vi "RunTest.vi"(8 "error in":errorcluster, 11 "Prueba31 in":refnum<class "Prueba32.lvclass">) -> (0 "error out":errorcluster, 2 "Resultado":string, 3 "Prueba31 out":refnum<class "Prueba32.lvclass">)   [LabVIEW 2019, in "Prueba32.lvclass"]
uses:
  Prueba32.lvclass
  Prueba32.lvclass/Prueba32.ctl
  <vilib>/Utility/miscctls.llb/LVRowAndColumnTypeDef.ctl
  QMH/Message Queue/Enqueue Message (Single).vi
  <vilib>/Utility/error.llb/Error Cluster From Error Code.vi
  RerenceAllControlsToolkit/_get control reference by name.vi
  <vilib>/ErrorRing/Error Ring.xnode
  QMH/Message Queue/Message Queue.lvlib
  QMH/User Event - Stop/User Event - Stop.lvlib
panel:
  in  "Tab":enum32{"externo", "interno"}(tab)
  out "Pict RingB_Ext":u16(ring)
  out "curva_referencia_Ext":dbl
  in  "cb_frec_Ext":string(combo)="63"
  in  "boton_generar_Ext":bool
  out "cumple_Ext":bool
  out "no_cumple_Ext":bool
  in  "seguir_Ext":bool
  out "voltaje_Ext":dbl format="%_3f"
  out "frecuencia_Ext":dbl format="%.2f"
  out "tipo generador_Ext":string
  out "Pict RingA_Ext":u16(ring)
  in  "Tabla_Ext":string[][](table)=[["63"], ["125"], ["250"], ["500"], ["1000"], ["2000"], ["4000"], ["8000"]]
  out "cumple_Int":bool
  out "no_cumple_Int":bool
  in  "seguir_Int":bool
  out "tipo generador_Int":string
  out "Pict RingA_Int":u16(ring)
  out "Pict RingB_Int":u16(ring)
  in  "Tabla_Int":string[][](table)
  # "Cumple"
  # "No Cumple"
  # "Curva de Referencia"
  # "Frecuencia"
  # "2. Ponderación frecuencial A (entrada acústica). IEC 61252: 2002 Cláusula 7"
  # "Monitoreo"
  # "Frecuencia"
  # "Hz"
  # "Voltaje"
  # "V"
  # "Cumple"
  # "No Cumple"
  # "2. Ponderación frecuencial A (entrada acústica). IEC 61252: 2002 Cláusula 7"
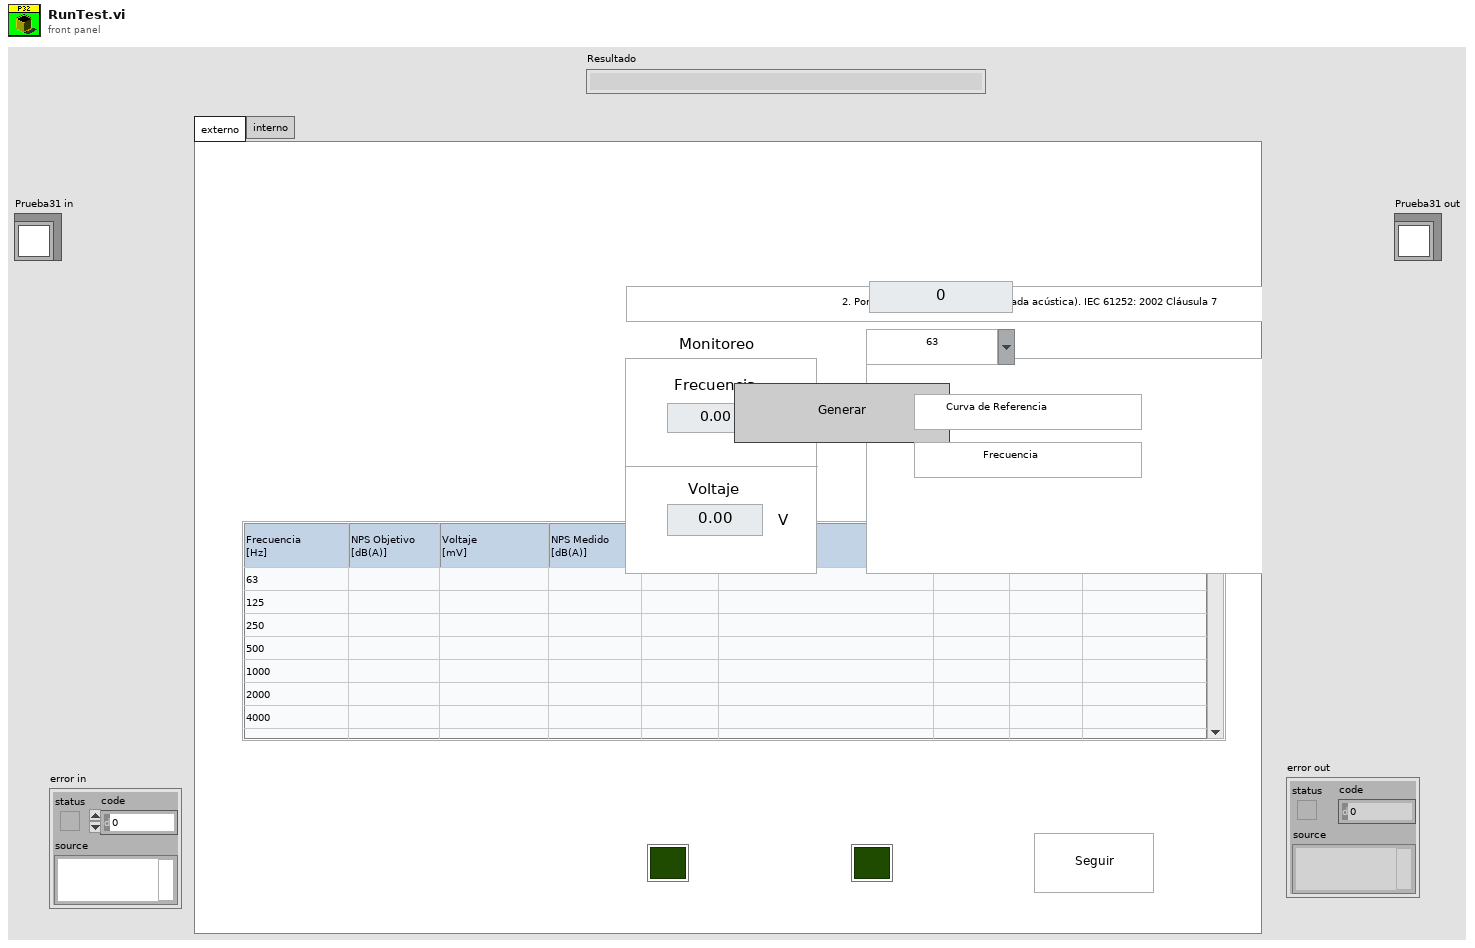
[diagram p1: front panel]
types:
  T1 = typedef "Message Queue.lvlib/All Message Queues.ctl" = cluster{"MHL":refnum<queue>, "Inst_CNT90":refnum<queue>, "Inst_DS360":refnum<queue>, "Inst_Keithley2002":refnum<queue>, "Inst_DAQ":refnum<queue>, "BD":refnum<queue>, "Pistofono":refnum<queue>, "Nexus":refnum<queue>}
  T2 = typedef "LVRowAndColumnTypeDef.ctl" = cluster{"Row":i32, "Column":i32}
  T3 = cluster{"ControlName":string, "ControlReference":refnum<vi>}[]
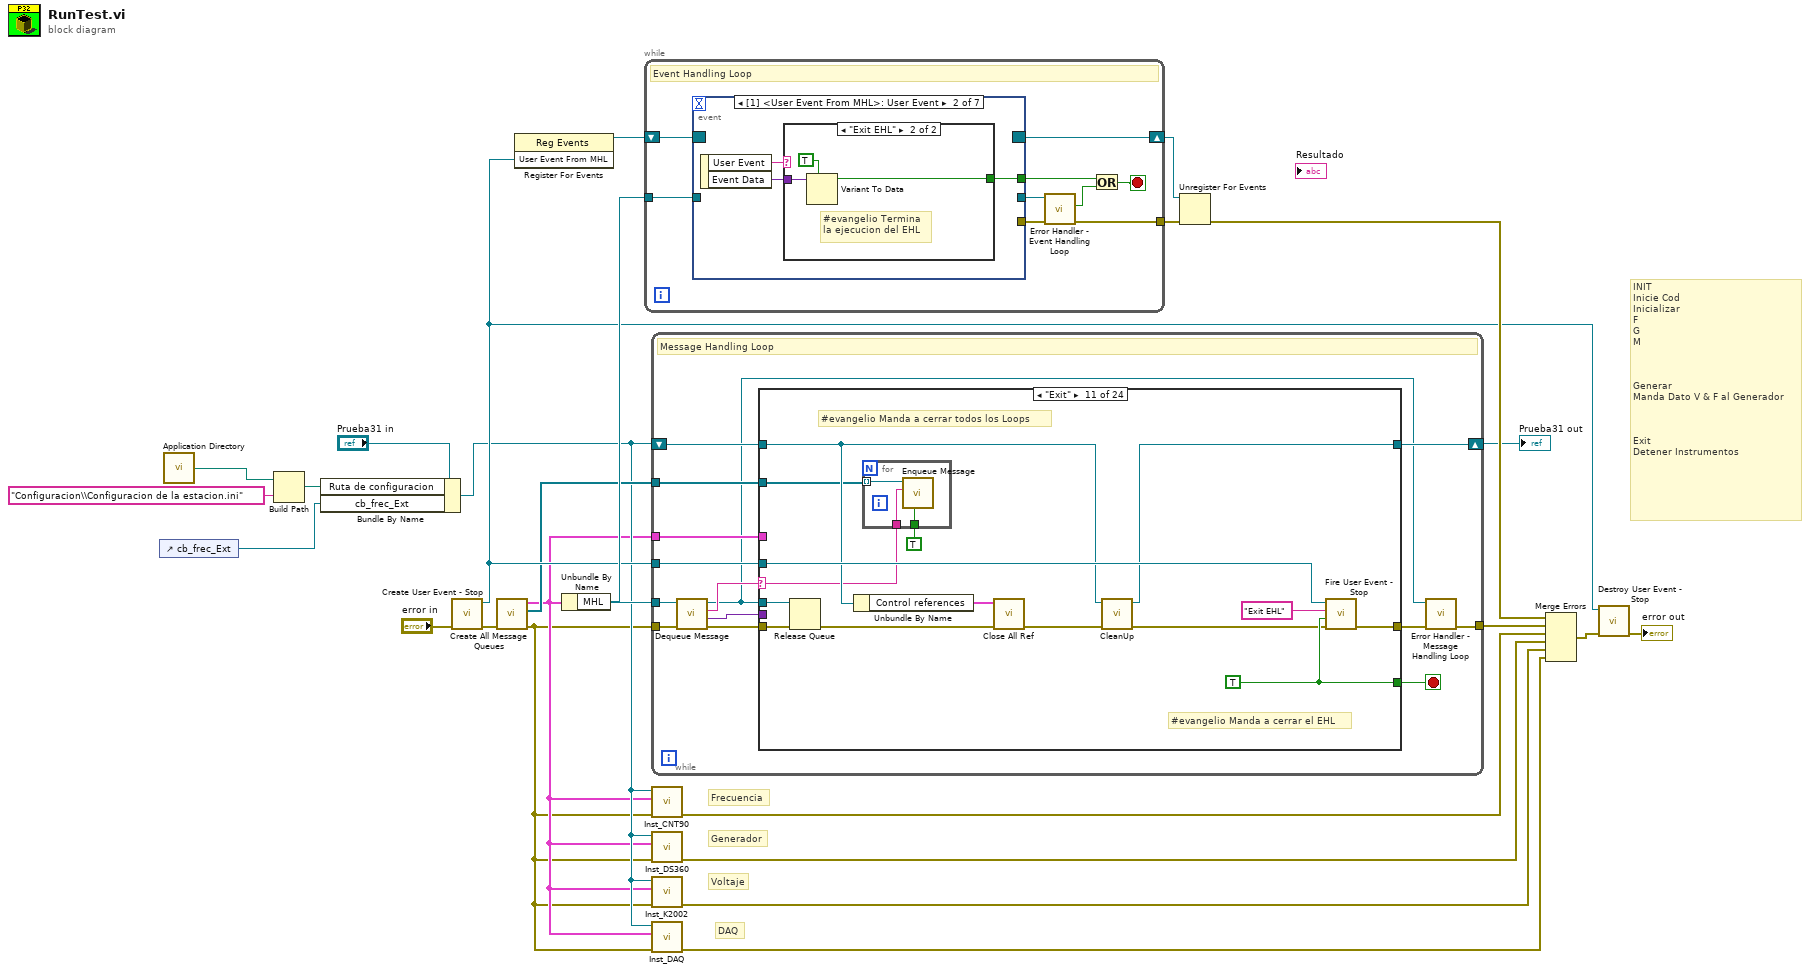
[diagram p0: block diagram]
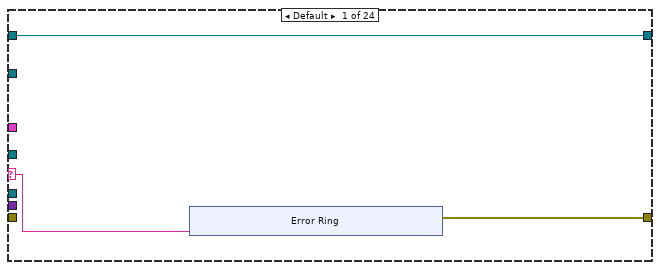
[diagram p2: hidden frame]
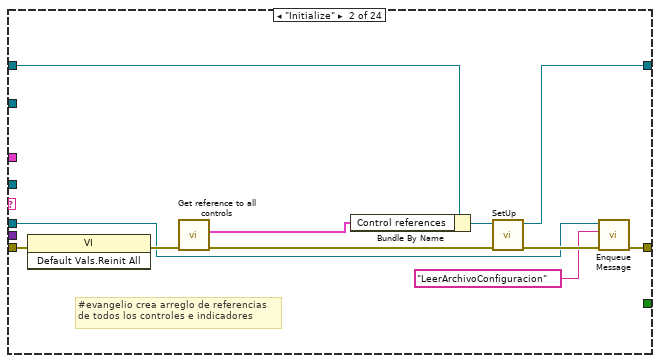
[diagram p3: hidden frame]
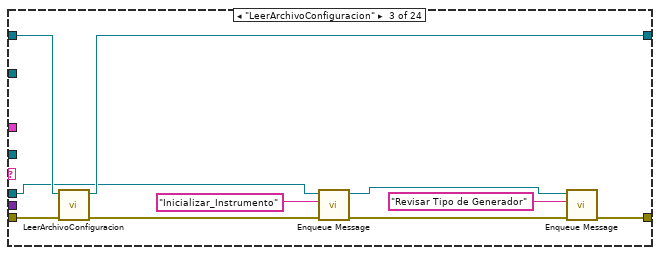
[diagram p4: hidden frame]
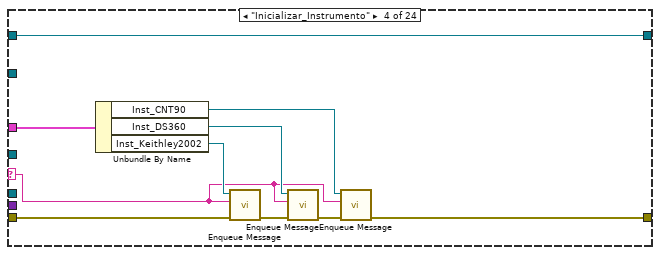
[diagram p5: hidden frame]
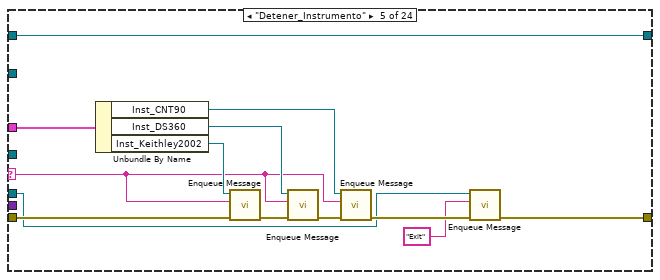
[diagram p6: hidden frame]
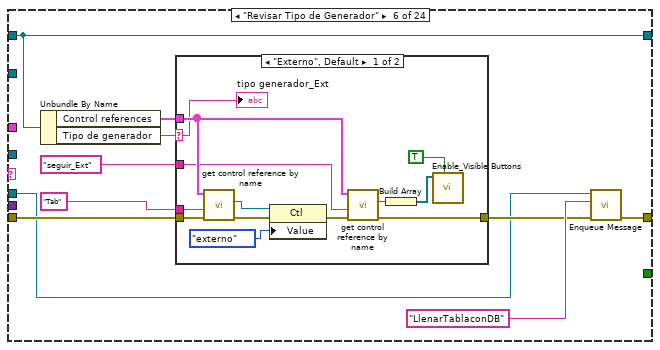
[diagram p7: hidden frame]
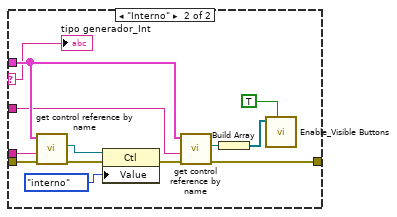
[diagram p8: hidden frame]
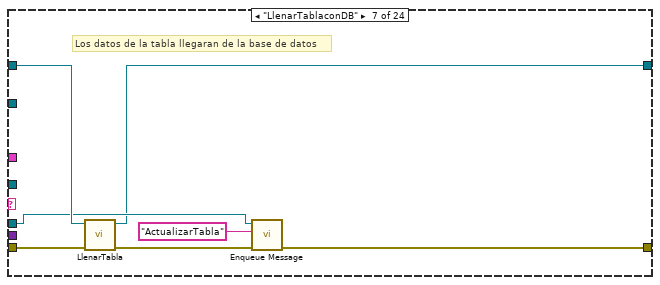
[diagram p9: hidden frame]
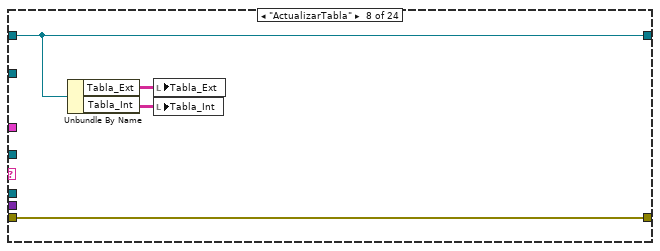
[diagram p10: hidden frame]
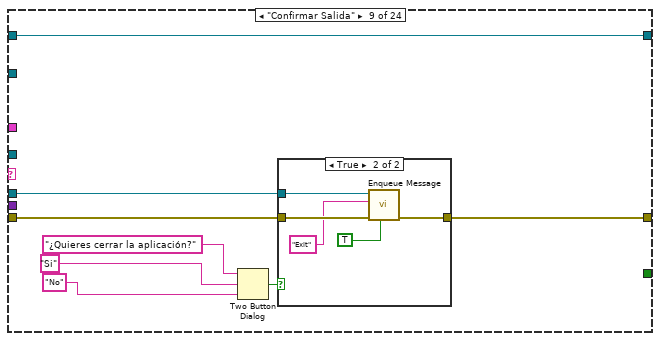
[diagram p11: hidden frame]
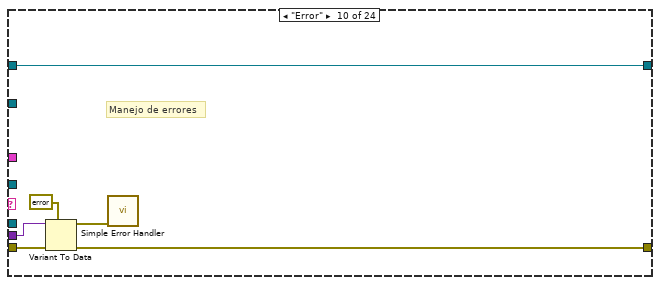
[diagram p13: hidden frame]
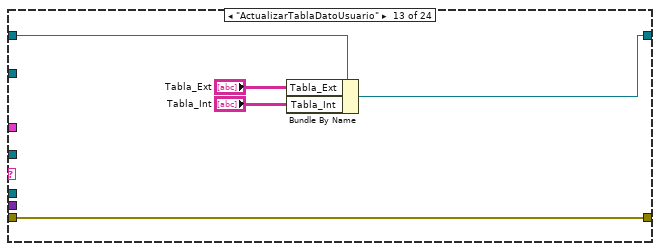
[diagram p15: hidden frame]
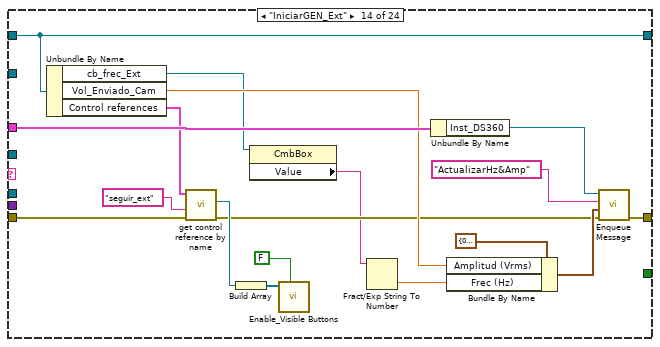
[diagram p16: hidden frame]
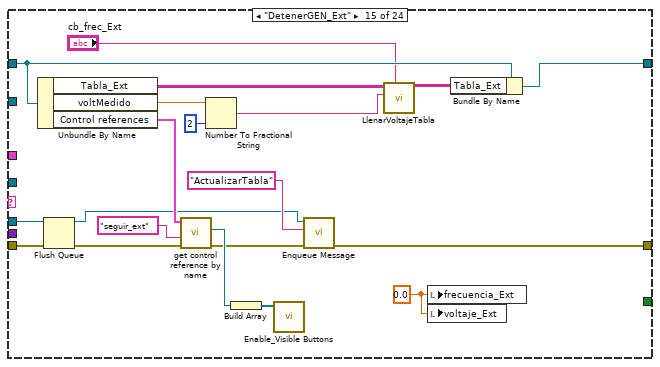
[diagram p17: hidden frame]
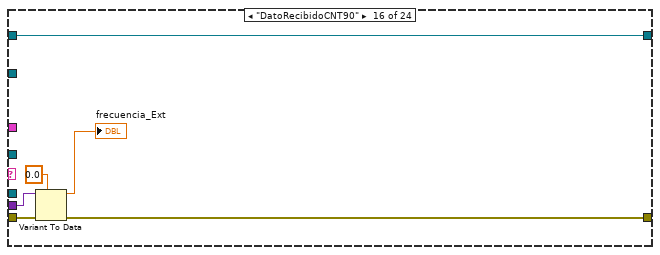
[diagram p18: hidden frame]
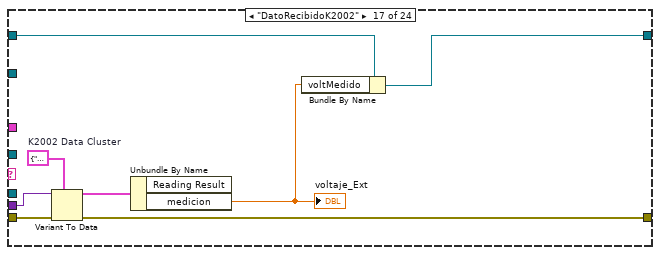
[diagram p19: hidden frame]
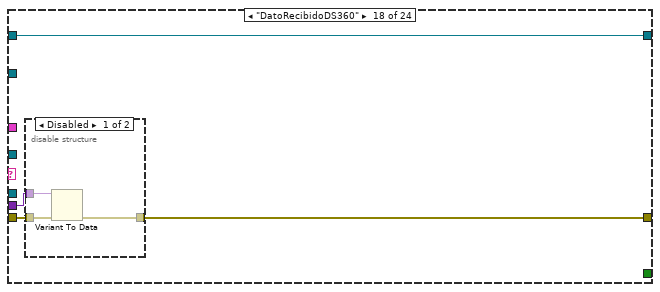
[diagram p20: hidden frame]
diagram:
  # "INIT\nInicie Cod\nInicializar\nF\nG\nM\n\n\n\nGenerar\nManda Dato V & F al Generador\n\n\n\nExit\nDetener Instrumentos"
  # "DAQ"
  # "Generador"
  # "Voltaje"
  # "Frecuencia"
  n1 = control-ref of="cb_frec_Ext"() -> (w1:refnum<vi>)
  n2 = call <vilib>:"Application Directory.vi"() -> ("Application Directory"=w9:path)
  n3 = Build Path(base path=w9, name or relative path="Configuracion\\Configuracion de la estacion.ini") -> (appended path=w8:path)
  n4 = Bundle By Name(cluster="Prueba31 in", "Ruta de configuracion"=w8, "cb_frec_Ext"=w1) -> (w5:refnum<class "Prueba32.lvclass">)
  n5 = call "Create User Event - Stop.vi"("error in (no error)"="error in") -> ("error out"=w22:errorcluster, "User Event From MHL"=w16:refnum<user-event>)  [unwired: 9 in]
  n6 = call "Create All Message Queues.vi"("error in (no error)"=w22) -> ("error out"=w3:errorcluster, "PL Queues Array"=w6:refnum<queue>[], "All Message Queues out"=w4:T1)  [unwired: 8 in]
  n7 = register-events(w16) -> (reference out=w25:refnum<event-registration>)  [unwired: 2 in, 1 out]
  n8 = Unbundle By Name(w4) -> ("MHL"=w21:refnum<queue>)
  n9 = while {
    tunnel: w21 -> [w34]
    tunnel: [w30] -> w24
    shift-right: [w32] -> w23
    shift-left: w25 -> [w33]
    stop <- w26 stop-if-true
    # "Event Handling Loop"
    n10 = event shown="[1] <User Event From MHL>: User Event" {
      selector: w33 -> [_ _ _ _ _ _ _]
      dyn-events: [_ _ _ _ _ _ _] -> w32
      timeout: _ -> [_ _ _ _ _ _ _]
      tunnel: w34 -> [w37 _ w47 w54 w58 w68 w71]
      tunnel: [w39 _ w48 w56 w63 w69 w72] -> w31
      tunnel: [w38 _ _ _ _ _ _] -> w29
      tunnel: [_ w40 _ _ _ _ _] -> w27
      event Panel Close? {
        w35 = TRUE
        n11 = event-data() -> ()  [unwired: 1 in, 1 out]
        n12 = call-poly "Enqueue Message.vi"("Priority Message? (F)"=w35, "Message"="Confirmar Salida", "Message Queue"=w37) -> ("error out"=w39:errorcluster, "dup Message Queue"=w38:refnum<queue>)  [unwired: 7 in]
        n13 = event-data("Discard?"=w35) -> ()  [unwired: 1 in, 1 out]
      }
      event User Event {
        n14 = event-data() -> ("User Event"=w42:string, "Event Data"=w41:variant)  [unwired: 1 in]
        n15 = case shown="\"Exit EHL\"" w42 {
          tunnel: w41 -> [_ w44]
          tunnel: [_ w43] -> w40
          frame Default {
          }
          frame "Exit EHL" {
            # "#evangelio Termina\nla ejecucion del EHL"
            n16 = Variant To Data(type=TRUE, Variant=w44) -> (data=w43:bool)  [unwired: 1 in, 1 out]
          }
        }
      }
      event "seguir_Ext", "seguir_Int": Value Change {
        n17 = event-data() -> ()  [unwired: 1 in, 1 out]
        n18 = call-poly "Enqueue Message.vi"("Message"="Detener_Instrumento", "Message Queue"=w47) -> ("error out"=w48:errorcluster)  [unwired: 8 in, 1 out]
      }
      event "Tabla_Ext": Value Change {
        n19 = event-data() -> ("CtlRef"=w50:refnum<vi>)  [unwired: 1 in]
        n20 = property class="Tbl (strict)"(reference=w50) -> ("Selection Start"=w49:T2)  [unwired: 1 in, 2 out]
        n21 = call-poly "Enqueue Message.vi"("Message"="ActualizarTablaDatoUsuario", "Message Queue"=w54) -> ("error out"=w51:errorcluster, "dup Message Queue"=w53:refnum<queue>)  [unwired: 8 in]
        n22 = call-poly "Enqueue Message.vi"("error in (no error)"=w51, "Message Data"=w49, "Message"="Evaluacion", "Message Queue"=w53) -> ("error out"=w56:errorcluster)  [unwired: 6 in, 1 out]
      }
      event "Tabla_Int": Value Change {
        n23 = event-data() -> ()  [unwired: 1 in, 2 out]
        n24 = property on="Tabla_Int" class="Tbl (strict)"() -> ("Selection Start"=w61:T2)  [unwired: 2 in, 2 out]
        n25 = call-poly "Enqueue Message.vi"("Message"="ActualizarTablaDatoUsuario", "Message Queue"=w58) -> ("error out"=w60:errorcluster, "dup Message Queue"=w59:refnum<queue>)  [unwired: 8 in]
        n26 = call-poly "Enqueue Message.vi"("error in (no error)"=w60, "Message Data"=w61, "Message"="Evaluacion", "Message Queue"=w59) -> ("error out"=w63:errorcluster)  [unwired: 6 in, 1 out]
      }
      event "boton_generar_Ext": Value Change {
        n27 = event-data() -> ()  [unwired: 1 in, 1 out]
        n28 = Select(t="IniciarGEN_Ext" ("Message"), s="boton_generar_Ext", f="DetenerGEN_Ext" ("Message")) -> (s? t:f=w66:string)
        n29 = call-poly "Enqueue Message.vi"("Message"=w66, "Message Queue"=w68) -> ("error out"=w69:errorcluster)  [unwired: 8 in, 1 out]
      }
      event "cb_frec_Ext": Value Change {
        n30 = event-data() -> ()  [unwired: 1 in, 1 out]
        n31 = call-poly "Enqueue Message.vi"("Message"="ActualizarCurvaRef", "Message Queue"=w71) -> ("error out"=w72:errorcluster)  [unwired: 8 in, 1 out]
      }
    }
    n32 = call "Error Handler - Event Handling Loop.vi"("error in (no error)"=w31, "Message Queue"=w29) -> ("dup error in"=w30:errorcluster, "Error?"=w28:bool)  [unwired: 7 in, 1 out]
    n33 = Or(x=w27, y=w28) -> (x .or. y?=w26:bool)
  }
  n34 = while {
    tunnel: w3 -> [w86]
    tunnel: w21 -> [w85]
    tunnel: [w80] -> w19
    shift-right: [w78] -> w17
    shift-left: w5 -> [w79]
    tunnel: w4 -> [w76]
    tunnel: w16 -> [w75]
    tunnel: w6 -> [w74]
    stop <- w77 stop-if-true
    # "Message Handling Loop"
    n35 = call "Dequeue Message.vi"("error in (no error)"=w86, "Message Queue"=w85) -> ("error out"=w82:errorcluster, "Message Data"=w83:variant, "Message"=w84:string, "dup Message Queue"=w73:refnum<queue>)  [unwired: 6 in]
    n36 = case shown="\"Exit\"" w84 {
      selector: w84 -> [w88 _ _ w121 w134 _ _ _ _ _ w210 _ _ _ _ _ _ _ w293 w303 _ _ _ _]
      tunnel: w73 -> [_ w100 w113 _ w129 w141 w180 _ w188 _ w221 _ _ _ w253 _ _ _ _ _ w316 _ _ _]
      tunnel: w83 -> [_ _ _ _ _ _ _ _ _ w203 _ _ _ _ _ w273 w282 w285 w300 w310 w325 _ _ _]
      tunnel: w82 -> [_ w107 w117 w126 w139 w147 w183 w187 w194 w204 w220 w227 w232 w243 w255 w274 w283 w286 w301 w311 w326 w335 w337 w339]
      tunnel: [w87 w101 w108 w118 w130 w142 w177 w187 w193 w205 w218 w227 w232 w241 w251 w275 w284 w287 w297 w307 w317 w335 w337 w339] -> w81
      tunnel: w79 -> [w89 w105 w116 w127 w140 w146 w182 w186 w195 w207 w211 w226 w230 w244 w262 w276 w277 w288 w302 w312 w321 w334 w336 w338]
      tunnel: [w89 w103 w115 w127 w140 w146 w178 w186 w195 w207 w212 w226 w231 w244 w263 w276 w278 w288 w302 w312 w314 w334 w336 w338] -> w78
      tunnel: [_ _ _ _ _ _ _ _ _ _ w215 _ _ _ _ _ _ _ _ _ _ _ _ _] -> w77
      tunnel: w76 -> [_ _ _ w125 w138 _ _ _ _ _ _ _ _ w250 _ _ _ _ w295 w305 _ _ _ _]
      tunnel: w75 -> [_ _ _ _ _ _ _ _ _ _ w217 _ _ _ _ _ _ _ _ _ _ _ _ _]
      tunnel: w74 -> [_ _ _ _ _ _ _ _ _ _ w208 _ _ _ _ _ _ _ _ _ _ _ _ _]
      frame Default {
        n37 = xnode "Error Ring"("parameter 0"=w88) -> ("error out"=w87:errorcluster)
      }
      frame "Initialize" {
        # "#evangelio crea arreglo de referencias\nde todos los controles e indicadores"
        n38 = invoke class="VI" method="Default Vals.Reinit All"(error in=w107) -> (error out=w106:errorcluster)  [unwired: 2 in, 2 out]
        n39 = call "Get reference to all controls.vi"("error in (no error)"=w106) -> ("error out"=w97:errorcluster, "Control references"=w98:T3)  [unwired: 5 in]
        n40 = Bundle By Name(cluster=w105, "Control references"=w98) -> (w104:refnum<class "Prueba32.lvclass">)
        n41 = call-dynamic "SetUp.vi"("error in (no error)"=w97, "Prueba08 in"=w104) -> ("error out"=w102:errorcluster, "Prueba08 out"=w103:refnum<class "Prueba32.lvclass">)  [unwired: 8 in]
        n42 = call-poly "Enqueue Message.vi"("error in (no error)"=w102, "Message"="LeerArchivoConfiguracion", "Message Queue"=w100) -> ("error out"=w101:errorcluster)  [unwired: 7 in, 1 out]
      }
      frame "LeerArchivoConfiguracion" {
        n43 = call "LeerArchivoConfiguracion.vi"("error in"=w117, "Prueba31 in"=w116) -> ("error out"=w114:errorcluster, "Prueba31 out"=w115:refnum<class "Prueba32.lvclass">)  [unwired: 8 in]
        n44 = call-poly "Enqueue Message.vi"("error in (no error)"=w114, "Message"="Inicializar_Instrumento", "Message Queue"=w113) -> ("error out"=w109:errorcluster, "dup Message Queue"=w110:refnum<queue>)  [unwired: 7 in]
        n45 = call-poly "Enqueue Message.vi"("error in (no error)"=w109, "Message"="Revisar Tipo de Generador", "Message Queue"=w110) -> ("error out"=w108:errorcluster)  [unwired: 7 in, 1 out]
      }
      frame "Inicializar_Instrumento" {
        n46 = Unbundle By Name(w125) -> ("Inst_CNT90"=w122:refnum<queue>, "Inst_DS360"=w123:refnum<queue>, "Inst_Keithley2002"=w124:refnum<queue>)
        n47 = call-poly "Enqueue Message.vi"("error in (no error)"=w126, "Message"=w121, "Message Queue"=w124) -> ("error out"=w120:errorcluster)  [unwired: 7 in, 1 out]
        n48 = call-poly "Enqueue Message.vi"("error in (no error)"=w120, "Message"=w121, "Message Queue"=w123) -> ("error out"=w119:errorcluster)  [unwired: 7 in, 1 out]
        n49 = call-poly "Enqueue Message.vi"("error in (no error)"=w119, "Message"=w121, "Message Queue"=w122) -> ("error out"=w118:errorcluster)  [unwired: 7 in, 1 out]
      }
      frame "Detener_Instrumento" {
        n50 = Unbundle By Name(w138) -> ("Inst_CNT90"=w135:refnum<queue>, "Inst_DS360"=w136:refnum<queue>, "Inst_Keithley2002"=w137:refnum<queue>)
        n51 = call-poly "Enqueue Message.vi"("error in (no error)"=w139, "Message"=w134, "Message Queue"=w137) -> ("error out"=w133:errorcluster)  [unwired: 7 in, 1 out]
        n52 = call-poly "Enqueue Message.vi"("error in (no error)"=w133, "Message"=w134, "Message Queue"=w136) -> ("error out"=w132:errorcluster)  [unwired: 7 in, 1 out]
        n53 = call-poly "Enqueue Message.vi"("error in (no error)"=w132, "Message"=w134, "Message Queue"=w135) -> ("error out"=w131:errorcluster)  [unwired: 7 in, 1 out]
        n54 = call-poly "Enqueue Message.vi"("error in (no error)"=w131, "Message"="Exit", "Message Queue"=w129) -> ("error out"=w130:errorcluster)  [unwired: 7 in, 1 out]
      }
      frame "Revisar Tipo de Generador" {
        n55 = Unbundle By Name(w146) -> ("Control references"=w149:T3, "Tipo de generador"=w150:string)
        n56 = case shown="\"Externo\", Default" w150 {
          selector: w150 -> [w151 w164]
          tunnel: w147 -> [w163 w176]
          tunnel: w149 -> [w158 w171]
          tunnel: "Tab" -> [w162 w175]
          tunnel: "seguir_Ext" -> [w156 w169]
          tunnel: [w153 w166] -> w143
          frame "Externo", Default {
            n57 = call-poly "get control reference by name.vi"("error in (no error)"=w163, "Control name"=w162, "Control references"=w158) -> ("error out"=w160:errorcluster, "Ctl Refnum"=w161:refnum<vi>)  [unwired: 3 in]
            n58 = property class="Ctl"(reference=w161, error in=w160, "Value"=enum32{"externo", "interno"}."externo" ("Tab Control")) -> (error out=w157:errorcluster)  [unwired: 1 out]
            n59 = call-poly "get control reference by name.vi"("error in (no error)"=w157, "Control name"=w156, "Control references"=w158) -> ("error out"=w153:errorcluster, "Ctl Refnum"=w155:refnum<vi>)  [unwired: 3 in]
            n60 = Build Array(w155) -> (w154:refnum<vi>[])
            n61 = call "Enable_Visible Buttons.vi"("Enable? (T)"=TRUE, "Controls Ref Array"=w154) -> ()  [unwired: 10 in]
            "tipo generador_Ext" <- w151
          }
          frame "Interno" {
            n62 = call-poly "get control reference by name.vi"("error in (no error)"=w176, "Control name"=w175, "Control references"=w171) -> ("error out"=w173:errorcluster, "Ctl Refnum"=w174:refnum<vi>)  [unwired: 3 in]
            n63 = property class="Ctl"(reference=w174, error in=w173, "Value"=enum32{"externo", "interno"}."interno" ("Tab Control")) -> (error out=w170:errorcluster)  [unwired: 1 out]
            n64 = call-poly "get control reference by name.vi"("error in (no error)"=w170, "Control name"=w169, "Control references"=w171) -> ("error out"=w166:errorcluster, "Ctl Refnum"=w168:refnum<vi>)  [unwired: 3 in]
            n65 = Build Array(w168) -> (w167:refnum<vi>[])
            n66 = call "Enable_Visible Buttons.vi"("Enable? (T)"=TRUE, "Controls Ref Array"=w167) -> ()  [unwired: 10 in]
            "tipo generador_Int" <- w164
          }
        }
        n67 = call-poly "Enqueue Message.vi"("error in (no error)"=w143, "Message"="LlenarTablaconDB", "Message Queue"=w141) -> ("error out"=w142:errorcluster)  [unwired: 7 in, 1 out]
      }
      frame "LlenarTablaconDB" {
        # "Los datos de la tabla llegaran de la base de datos"
        n68 = call "LlenarTabla.vi"("error in (no error)"=w183, "Prueba32 in"=w182) -> ("error out"=w181:errorcluster, "Prueba32 out"=w178:refnum<class "Prueba32.lvclass">)  [unwired: 8 in]
        n69 = call-poly "Enqueue Message.vi"("error in (no error)"=w181, "Message"="ActualizarTabla", "Message Queue"=w180) -> ("error out"=w177:errorcluster)  [unwired: 7 in, 1 out]
      }
      frame "ActualizarTabla" {
        n70 = Unbundle By Name(w186) -> ("Tabla_Ext"=w185:string[][], "Tabla_Int"=w184:string[][])
        n71 = local write "Tabla_Ext"(w185) -> ()
        n72 = local write "Tabla_Int"(w184) -> ()
      }
      frame "Confirmar Salida" {
        n73 = Two Button Dialog(message="¿Quieres cerrar la aplicación?", 1:"No" ("T button name (\"OK\")"), 2:"Si" ("T button name (\"OK\")")) -> (T button?=w189:bool)
        n74 = case shown="True" w189 {
          tunnel: w194 -> [w196 w201]
          tunnel: [w196 w200] -> w193
          tunnel: w188 -> [_ w199]
          frame False {
          }
          frame True {
            n75 = call-poly "Enqueue Message.vi"("Priority Message? (F)"=TRUE, "error in (no error)"=w201, "Message"="Exit", "Message Queue"=w199) -> ("error out"=w200:errorcluster)  [unwired: 6 in, 1 out]
          }
        }
      }
      frame "Error" {
        # "Manejo de errores"
        n76 = Variant To Data(error in=w204, type=errorcluster {"status"=FALSE, "code"=0, "source"=""} ("error constant"), Variant=w203) -> (data=w202:errorcluster, error out=w205:errorcluster)
        n77 = call <vilib>:"Simple Error Handler.vi"("error in (no error)"=w202) -> ()  [unwired: 4 in, 5 out]
      }
      frame "Exit" {
        w215 = TRUE
        # "#evangelio Manda a cerrar el EHL"
        # "#evangelio Manda a cerrar todos los Loops"
        n78 = Release Queue(queue=w221, error in (no error)=w220) -> (error out=w219:errorcluster)  [unwired: 1 in, 2 out]
        n79 = Unbundle By Name(w211) -> ("Control references"=w222:T3)
        n80 = for {
          tunnel: w208 -> [w225] mode=indexing
          tunnel: w210 -> [w224]
          tunnel: TRUE -> [w223]
          n81 = call-poly "Enqueue Message.vi"("Priority Message? (F)"=w223, "Message"=w224, "Message Queue"=w225) -> ()  [unwired: 7 in, 2 out]
        }
        n82 = call "Close All Ref.vi"("error in (no error)"=w219, "Control references"=w222) -> ("error out"=w214:errorcluster)  [unwired: 9 in]
        n83 = call-dynamic "CleanUp.vi"("error in (no error)"=w214, "Prueba08 in"=w211) -> ("error out"=w213:errorcluster, "Prueba08 out"=w212:refnum<class "Prueba32.lvclass">)  [unwired: 8 in]
        n84 = call "Fire User Event - Stop.vi"("error in (no error)"=w213, "Event Data"=w215, "User Event"="Exit EHL", "User Event in"=w217) -> ("error out"=w218:errorcluster)  [unwired: 7 in]
      }
      frame "---- EXT ----" {
      }
      frame "ActualizarTablaDatoUsuario" {
        n85 = Bundle By Name(cluster=w230, "Tabla_Ext"="Tabla_Ext", "Tabla_Int"="Tabla_Int") -> (w231:refnum<class "Prueba32.lvclass">)
      }
      frame "IniciarGEN_Ext" {
        n86 = Unbundle By Name(w244) -> ("cb_frec_Ext"=w235:refnum<vi>, "Vol_Enviado_Cam"=w238:dbl, "Control references"=w237:T3)
        n87 = call-poly "get control reference by name.vi"("error in (no error)"=w243, "Control name"="seguir_ext", "Control references"=w237) -> ("error out"=w236:errorcluster, "Ctl Refnum"=w246:refnum<vi>)  [unwired: 3 in]
        n88 = Build Array(w246) -> (w245:refnum<vi>[])
        n89 = property class="CmbBox"(reference=w235) -> ("Value"=w234:string)  [unwired: 1 in, 2 out]
        n90 = call "Enable_Visible Buttons.vi"("Enable? (T)"=FALSE, "Controls Ref Array"=w245) -> ()  [unwired: 10 in]
        n91 = Fract/Exp String To Number(string=w234) -> (number=w233:dbl)  [unwired: 3 in, 1 out]
        n92 = Unbundle By Name(w250) -> ("Inst_DS360"=w249:refnum<queue>)
        n93 = Bundle By Name(cluster=cluster{"Amplitud (Vrms)":dbl, "Frec (Hz)":dbl} {"Amplitud (Vrms)"=0.0, "Frec (Hz)"=0.0}, "Amplitud (Vrms)"=w238, "Frec (Hz)"=w233) -> (w239:cluster{"Amplitud (Vrms)":dbl, "Frec (Hz)":dbl})
        n94 = call-poly "Enqueue Message.vi"("error in (no error)"=w236, "Message Data"=w239, "Message"="ActualizarHz&Amp", "Message Queue"=w249) -> ("error out"=w241:errorcluster)  [unwired: 6 in, 1 out]
      }
      frame "DetenerGEN_Ext" {
        w252 = 0.0 ("frecuencia_Ext")
        n95 = Unbundle By Name(w262) -> ("Tabla_Ext"=w259:string[][], "voltMedido"=w266:dbl, "Control references"=w267:T3)
        n96 = Flush Queue(queue=w253, error in (no error)=w255) -> (queue out=w254:refnum<queue>, error out=w256:errorcluster)  [unwired: 1 out]
        n97 = call-poly "get control reference by name.vi"("error in (no error)"=w256, "Control name"="seguir_ext", "Control references"=w267) -> ("error out"=w261:errorcluster, "Ctl Refnum"=w269:refnum<vi>)  [unwired: 3 in]
        n98 = Number To Fractional String(number=w266, precision (6)=i16 2) -> (F-format string=w257:string)  [unwired: 2 in]
        n99 = Build Array(w269) -> (w268:refnum<vi>[])
        n100 = call "Enable_Visible Buttons.vi"("Controls Ref Array"=w268) -> ()  [unwired: 11 in]
        n101 = call-poly "Enqueue Message.vi"("error in (no error)"=w261, "Message"="ActualizarTabla" ("Control name"), "Message Queue"=w254) -> ("error out"=w251:errorcluster)  [unwired: 7 in, 1 out]
        n102 = call "LlenarVoltajeTabla.vi"("Frecuencia"="cb_frec_Ext", "Dato"=w257, "Tabla in"=w259) -> ("Tabla out"=w264:string[][])  [unwired: 8 in]
        n103 = local write "frecuencia_Ext"(w252) -> ()
        n104 = local write "voltaje_Ext"(w252) -> ()
        n105 = Bundle By Name(cluster=w262, "Tabla_Ext"=w264) -> (w263:refnum<class "Prueba32.lvclass">)
      }
      frame "DatoRecibidoCNT90" {
        n106 = Variant To Data(error in=w274, type=0.0, Variant=w273) -> (data=→"frecuencia_Ext":dbl, error out=w275:errorcluster)
      }
      frame "DatoRecibidoK2002" {
        w281 = cluster{"Reading Result":string, "medicion":dbl} {"Reading Result"="", "medicion"=0.0}  # K2002 Data Cluster
        n107 = Variant To Data(error in=w283, type=w281, Variant=w282) -> (data=w280:cluster{"Reading Result":string, "medicion":dbl}, error out=w284:errorcluster)
        n108 = Unbundle By Name(w280) -> ("medicion"=w279:dbl)  [unwired: 1 out]
        "voltaje_Ext" <- w279
        n109 = Bundle By Name(cluster=w277, "voltMedido"=w279) -> (w278:refnum<class "Prueba32.lvclass">)
      }
      frame "DatoRecibidoDS360" {
        n110 = disable-structure shown="Disabled" {
          disable-tunnel: [w291 w292] -> w287
          disable-tunnel: w286 -> [w290 w292]
          disable-tunnel: w285 -> [w289 _]
          frame Disabled {
            n111 = Variant To Data(error in=w290, Variant=w289) -> (error out=w291:errorcluster)  [unwired: 1 in, 1 out]
          }
          frame Enabled {
          }
        }
      }
      frame "EnviarFrecuenciaRef" {
        n112 = Variant To Data(error in=w301, type=w293, Variant=w300) -> (data=w299:string, error out=w298:errorcluster)
        n113 = Unbundle By Name(w295) -> ("Inst_CNT90"=w294:refnum<queue>)
        n114 = Fract/Exp String To Number(string=w299) -> (number=w296:dbl)  [unwired: 3 in, 1 out]
        n115 = call-poly "Enqueue Message.vi"("error in (no error)"=w298, "Message Data"=w296, "Message"=w293, "Message Queue"=w294) -> ("error out"=w297:errorcluster)  [unwired: 6 in, 1 out]
      }
      frame "EnviarNivelRef" {
        n116 = Variant To Data(error in=w311, type=w303, Variant=w310) -> (data=w309:string, error out=w308:errorcluster)
        n117 = Unbundle By Name(w305) -> ("Inst_Keithley2002"=w304:refnum<queue>)
        n118 = Fract/Exp String To Number(string=w309) -> (number=w306:dbl)  [unwired: 3 in, 1 out]
        n119 = call-poly "Enqueue Message.vi"("error in (no error)"=w308, "Message Data"=w306, "Message"=w303, "Message Queue"=w304) -> ("error out"=w307:errorcluster)  [unwired: 6 in, 1 out]
      }
      frame "Evaluacion" {
        n120 = Variant To Data(error in=w326, type=T2 {"Row"=0, "Column"=0} ("Selection Start"), Variant=w325) -> (data=w323:T2, error out=w327:errorcluster)
        n121 = Unbundle By Name(w323) -> ("Row"=w320:i32, "Column"=w319:i32)
        n122 = call "ObtenerDatosdelatabla.vi"("Column"=w319, "Row"=w320, "Prueba32 in"=w321) -> ("Prueba32 out"=w322:refnum<class "Prueba32.lvclass">)  [unwired: 8 in]
        n123 = call "cumplimiento.vi"("error in (no error)"=w327, "Prueba08 in"=w322) -> ("error out"=w318:errorcluster, "Evaluarcion Final"=w313:bool, "Prueba08 out"=w314:refnum<class "Prueba32.lvclass">)  [unwired: 6 in, 1 out]
        n124 = call "EvaluacionFinal.vi"("Evaluacion Final"=w313, "Prueba32 in"=w314) -> ()  [unwired: 10 in]
        n125 = call-poly "Enqueue Message.vi"("error in (no error)"=w318, "Message"="ActualizarTabla", "Message Queue"=w316) -> ("error out"=w317:errorcluster)  [unwired: 7 in, 1 out]
      }
      frame "ActualizarCurvaRef" {
        n126 = Unbundle By Name(w334) -> ("Tabla_Ext"=w332:string[][])
        n127 = local read "cb_frec_Ext"() -> (w333:string)
        n128 = call "ObtenerFilaEnUso.vi"("Tabla in"=w332, "Frecuencia"=w333) -> ("index of element"=w331:i32)  [unwired: 9 in]
        n129 = Index Array(array=w332, index (row)=w331, index (col)=1 ("disabled index (col)")) -> (element=w329:string)
        n130 = Fract/Exp String To Number(string=w329) -> (number=→"curva_referencia_Ext":dbl)  [unwired: 3 in, 1 out]
      }
      frame "---- INT ----" {
      }
      frame "--------------------------Contoles---------------------------" {
      }
    }
    n131 = call "Error Handler - Message Handling Loop.vi"("error in (no error)"=w81, "Message Queue"=w73) -> ("dup error in"=w80:errorcluster)  [unwired: 8 in, 1 out]
  }
  "Prueba31 out" <- w17
  n132 = call "Inst_CNT90.vi"("error in"=w3, "All Message Queues in"=w4, "AjustesPrevios in"=w5) -> ("error out"=w13:errorcluster)  [unwired: 8 in]
  n133 = call "Inst_DS360.vi"("error in"=w3, "All Message Queues in"=w4, "Prueba31 in"=w5) -> ("error out"=w12:errorcluster)  [unwired: 8 in]
  n134 = call "Inst_K2002.vi"("error in"=w3, "All Message Queues in"=w4, "Prueba31 in"=w5) -> ("error out"=w11:errorcluster)  [unwired: 8 in]
  n135 = call "Inst_DAQ.vi"("error in"=w3, "All Message Queues in"=w4, "Prueba31 in"=w5) -> ("error out"=w2:errorcluster)  [unwired: 8 in]
  n136 = Unregister For Events(event registration refnum=w23, error in=w24) -> (error out=w20:errorcluster)
  n137 = Merge Errors(w20, w19, w13, w12, w11, w2) -> (w18:errorcluster)
  n138 = call "Destroy User Event - Stop.vi"("error in (no error)"=w18, "User Event"=w16) -> ("error out"=→"error out":errorcluster)  [unwired: 9 in]
